vi "PH_SSAC.evt call set Frame.vi"(0 "i ref in":refnum<vi>, 1 "Instance":string, 2 "Signal":T1, 3 "x":u32, 4 "dx":u32, 5 "error in":errorcluster, 7 "y":u32, 9 "dy":u32) -> (14 "i ref out":refnum<vi>, 19 "error out":errorcluster)   [LabVIEW 2014, in "PH_SSAC.lvlib"]
doc: "This VI calls an event case by a simple call."
uses:
  PH_SSAC.lvlib
  PH_SSAC.Signal Selector.ctl
  CSCore/CSSystem/CoreLib/CoreLib.int 2 byte array.vi
  CSCore/CSSystem/CoreLib/CoreLib.lvlib
  CSCore/BaseProcess/BaseProcess.lvlib
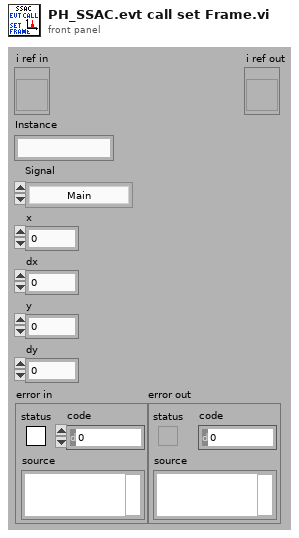
[diagram p1: front panel]
types:
  T1 = typedef "PH_SSAC.lvlib/PH_SSAC.Signal Selector.ctl" = enum16{"Main", "Background"}
  T2 = typedef "CoreDefs.rawDataType.ctl" = i8[]
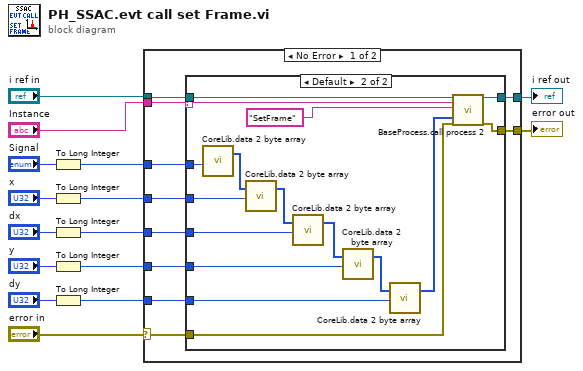
[diagram p0: block diagram]
diagram:
  n1 = To Long Integer(number="Signal") -> (32bit integer=w8:i32)
  n2 = To Long Integer(number="x") -> (32bit integer=w4:i32)
  n3 = To Long Integer(number="dx") -> (32bit integer=w3:i32)
  n4 = To Long Integer(number="y") -> (32bit integer=w2:i32)
  n5 = To Long Integer(number="dy") -> (32bit integer=w1:i32)
  n6 = case shown="No Error" "error in" {
    selector: "error in" -> [w22 w44]
    tunnel: [w25 w45] -> w13
    tunnel: [w24 w44] -> w12
    tunnel: "i ref in" -> [w23 w45]
    tunnel: "Instance" -> [w21 _]
    tunnel: w8 -> [w20 _]
    tunnel: w4 -> [w19 _]
    tunnel: w3 -> [w18 _]
    tunnel: w2 -> [w17 _]
    tunnel: w1 -> [w16 _]
    frame No Error {
      n7 = case shown="Default" w21 {
        selector: w21 -> [_ w28]
        tunnel: [w27 w42] -> w25
        tunnel: [w26 w41] -> w24
        tunnel: w23 -> [w27 w40]
        tunnel: w22 -> [w26 w39]
        tunnel: w20 -> [_ w38]
        tunnel: w19 -> [_ w35]
        tunnel: w18 -> [_ w33]
        tunnel: w17 -> [_ w32]
        tunnel: w16 -> [_ w30]
        frame "N/A" {
        }
        frame Default {
          n8 = call-poly "CoreLib.data 2 byte array.vi"("i32"=w38) -> ("byteArray out"=w37:T2)  [unwired: 18 in]
          n9 = call-poly "CoreLib.data 2 byte array.vi"("byteArray"=w37, "i32"=w35) -> ("byteArray out"=w34:T2)  [unwired: 17 in]
          n10 = call-poly "CoreLib.data 2 byte array.vi"("byteArray"=w34, "i32"=w33) -> ("byteArray out"=w36:T2)  [unwired: 17 in]
          n11 = call-poly "CoreLib.data 2 byte array.vi"("byteArray"=w36, "i32"=w32) -> ("byteArray out"=w31:T2)  [unwired: 17 in]
          n12 = call-poly "CoreLib.data 2 byte array.vi"("byteArray"=w31, "i32"=w30) -> ("byteArray out"=w29:T2)  [unwired: 17 in]
          n13 = call "BaseProcess.call process 2.vi"("i ref in"=w40, "Object"=w28, "Selector"="SetFrame", "Data"=w29, "error in (no error)"=w39) -> ("i ref out"=w42:refnum<vi>, "error out"=w41:errorcluster)  [unwired: 13 in]
        }
      }
    }
    frame Error {
    }
  }
  "i ref out" <- w13
  "error out" <- w12
